vi "Copy File.vi"(7 "overwrite":bool, 8 "error in (no error)":errorcluster caption="错误输入（无错误）", 9 "DestinationFileName":path, 10 "SourceFileName":path, 11 "FileSystem 输入":refnum<class "FileSystem.lvclass"> caption="DNL_LabVIEW Object in") -> (0 "error out":errorcluster caption="错误输出", 3 "FileSystem 输出":refnum<class "FileSystem.lvclass"> caption="DNL_LabVIEW Object out")   [LabVIEW 2012, in "FileSystem.lvclass"]
uses:
  FileSystem.lvclass
  FileSystem.lvclass/FileSystem.ctl
  Microsoft.VisualBasic
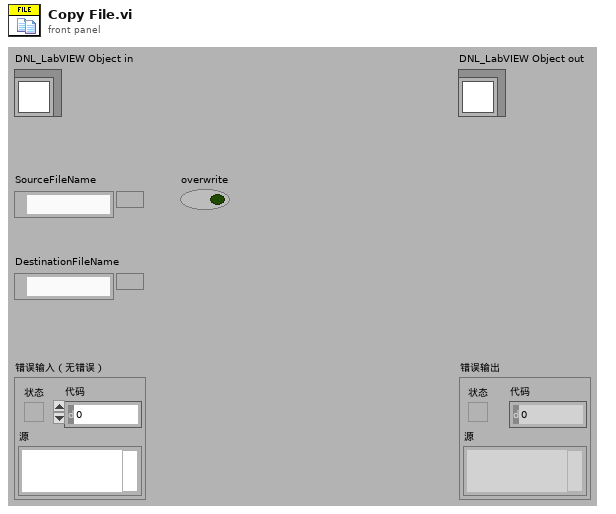
[diagram p1: front panel]
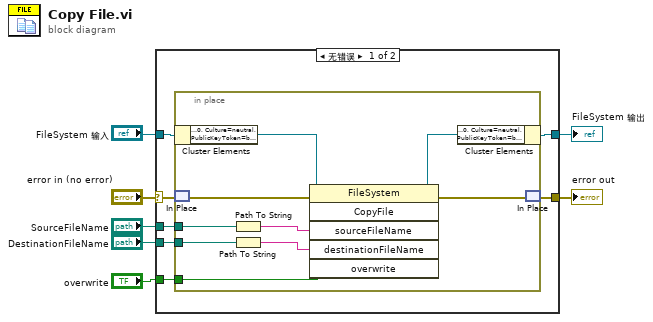
[diagram p0: block diagram]
diagram:
  n1 = case shown="无错误" "error in (no error)" {
    selector: "error in (no error)" -> [w13 w25]
    tunnel: [w12 w25] -> w6
    tunnel: [w8 w24] -> w4
    tunnel: "FileSystem 输入" -> [w14 w24]
    tunnel: "overwrite" -> [w11 _]
    tunnel: "SourceFileName" -> [w10 _]
    tunnel: "DestinationFileName" -> [w9 _]
    frame No Error {
      n2 = in-place {
        in-place-border: w11 -> [w19]
        in-place-border: w10 -> [w18]
        in-place-border: w9 -> [w16]
        n3 = in-place-cluster #1(w14) -> ("FileSystem"=w23:refnum<k24>)
        n4 = in-place-match #2(w13) -> (w21:errorcluster)
        n5 = Path To String(path=w18) -> (string=w17:string)
        n6 = Path To String(path=w16) -> (string=w15:string)
        n7 = invoke class="FileSystem" method="CopyFile"(reference=w23, error in=w21, "sourceFileName"=w17, "destinationFileName"=w15, "overwrite"=w19) -> (reference out=w22:refnum<k24>, error out=w20:errorcluster)  [unwired: 1 in, 4 out]
        n8 = in-place-cluster #1("FileSystem"=w22) -> (w8:refnum<class "FileSystem.lvclass">)
        n9 = in-place-match #2(w20) -> (w12:errorcluster)
      }
    }
    frame Error {
    }
  }
  "error out" <- w6
  "FileSystem 输出" <- w4
